vi "INIT_Q.vi"() -> (4 "MainQ Out":refnum<queue>, 6 "ACKQ Out":refnum<queue>, 8 "TempQ Out":refnum<queue>, 10 "MagQ Out":refnum<queue>, 15 "ScanQ Out":refnum<queue>)   [LabVIEW 2025]
uses:
  CTLs/Producer Cluster.ctl
  CTLs/ACK Cluster.ctl
  CTLs/TEMP CLUSTER.ctl
  CTLs/MAG CLUSTER.ctl
  CTLs/Scan Cluster.ctl
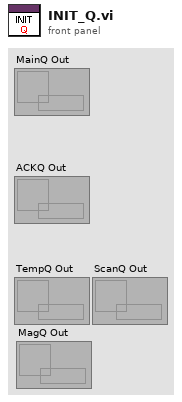
[diagram p1: front panel]
types:
  T1 = typedef "Scan Cluster.ctl" = cluster{"Setpoint (I)":dbl[], "Bias (V)":dbl[], "Number of scans":u8, "Port number (3364)":u32, "Avoid zero threshold (V)":dbl, "Current State":enum16{"1. BIAS", "2. SCAN", "3. SCAN_IDLE", "4. DRIFT CORRECT (SF)", "5. DRFT CORRECT (BS)", "6. STOP"}}
  T2 = typedef "MAG CLUSTER.ctl" = cluster{"Ramp Target":enum16{"ZERO", "MID", "MAX"}, "Pause":bool, "Switch Heater":bool, "Persistent Field":dbl, "Persistent Current":dbl, "Tesla":bool, "Output (T)":dbl, "Output (A)":dbl, "X Trip":enum16{"DISABLED", "ENABLED", "ACTIVE"}, "Ramp Rate (A/s)":dbl, "V Limit (V)":dbl, "Heater Voltage":dbl, "MAX Setpoint (A)":dbl, "MAX Setpoint (T)":dbl, "MID Setpoint (A)":dbl, "MID Setpoint (T)":dbl, "Lock":bool, "Field Constant":dbl, "Remote":bool, "Direction":enum16{"POSITIVE", "NEGATIVE", "OPEN", "UNIPOLAR"}, "Helium Level":u16, "Quench !":bool, "Voltage":dbl, "V Limit !":bool, "Ramping":bool, "At Target":bool, "Trip Field":dbl, "Trip Current":dbl, "Current State":enum16{"1. INIT MAG", "2. PREP FIELD", "3. APPLY FIELD", "4. MAG STAB", "5. MAG IDLE", "6. MAG OFF"}, "MAG Reference":refnum<visa-resource-name>}
  T3 = typedef "TEMP CLUSTER.ctl" = cluster{"Range (0:Off)":u16, "Manual Output (0.00 %)":dbl, "Rate (D) (0.0 %)":dbl, "Reset (I) (20.0)":dbl, "Gain (P) (50.0)":dbl, "Power Up Enable (F: Disable)":bool, "Max User Current (2.000)":dbl, "Heater Resistance (1:25 Ohms)":u16, "Max Current (0:User Specified)":u16, "Heater Out Display (1:Current)":u16, "Mode (0:Off)":u16, "Input (0:None)":u16, "Target Temp (K)":dbl, "Serial Configuration":cluster{"Baud Rate":u32, "Parity":u16, "Data Bits":u16, "Stop Bits":u16, "Flow Control":u16}, "VISA resource name":refnum<visa-resource-name>, "Configure Control Parameters (0: Configure)":u16, "Enable Setpoint (F:Disable)":bool, "Input (0:A)":u16, "Data Source (0:Kelvin)":u16, "Output's Control Loop (1:1)":u16, "STND DEV Threshold ":dbl, "Mean Tolerance ":dbl, "Current State":enum16{"1. INIT_TEMP", "2. SET_TEMP", "3. WAIT_STABLE", "4. TEMP_IDLE", "5. TC OFF (Reset)"}}
  T4 = typedef "ACK Cluster.ctl" = cluster{"ACK States":enum16{"1. TEMP STABLE", "2. FIELD STABLE", "3. SCAN DONE", "4. BIAS DONE", "5. DRIFT CORRECTED (SF)", "6. DRIFT CORRECTED (BS)"}, "Drift Correction Values":dbl[][]}
  T5 = typedef "Producer Cluster.ctl" = cluster{"Producer State":enum16{"1. INIT", "2. SET TEMP", "3. WAIT FOR STABILITY (T)", "4. SET FIELD ", "5. WAIT FOR STABILITY (B)", "6. RUN SCAN", "7. RUN BIAS", "8. DRIFT CORRECT (SF)", "9. DRIFT CORRECT (BS)", "10. ADVANCE", "11. SHUTDOWN"}, "Experiment Mode":enum16{"1. SWEEP FIELD", "2. SWEEP TEMP", "3. SWEEP FIELD AND TEMP"}, "Target Temp (K)":dbl[], "Target Field (T)":dbl[], "Temp Index":i32, "Field Index":i32, "Current Temp":dbl, "Current Field":dbl}
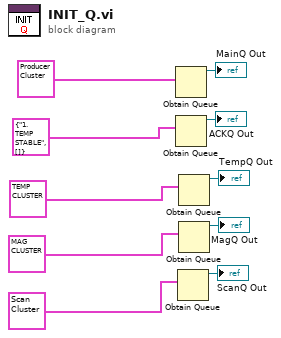
[diagram p0: block diagram]
diagram:
  n1 = Obtain Queue(element data type=T5 {"Producer State"=enum."1. INIT", "Experiment Mode"=enum."1. SWEEP FIELD", "Target Temp (K)"=[], "Target Field (T)"=[], "Temp Index"=0, "Field Index"=0, "Current Temp"=0.0, "Current Field"=0.0} ("Producer Cluster")) -> (queue out=→"MainQ Out":refnum<queue>)  [unwired: 4 in, 2 out]
  n2 = Obtain Queue(element data type=T4 {"ACK States"=enum."1. TEMP STABLE", "Drift Correction Values"=[]} ("ACK Cluster")) -> (queue out=→"ACKQ Out":refnum<queue>)  [unwired: 4 in, 2 out]
  n3 = Obtain Queue(element data type=T1 {"Setpoint (I)"=[], "Bias (V)"=[], "Number of scans"=1, "Port number (3364)"=3364, "Avoid zero threshold (V)"=0.004999999888241291, "Current State"=enum."1. BIAS"} ("Scan Parameters")) -> (queue out=→"ScanQ Out":refnum<queue>)  [unwired: 4 in, 2 out]
  n4 = Obtain Queue(element data type=T3 {"Range (0:Off)"=0, "Manual Output (0.00 %)"=0.0, "Rate (D) (0.0 %)"=0.0, "Reset (I) (20.0)"=20.0, "Gain (P) (50.0)"=50.0, "Power Up Enable (F: Disable)"=FALSE, "Max User Current (2.000)"=2.0, "Heater Resistance (1:25 Ohms)"=1, "Max Current (0:User Specified)"=0, "Heater Out Display (1:Current)"=1, "Mode (0:Off)"=1, "Input (0:None)"=4, "Target Temp (K)"=5.0, "Serial Configuration"={"Baud Rate"=57600, "Parity"=1, "Data Bits"=7, "Stop Bits"=10, "Flow Control"=0}, "VISA resource name"="", "Configure Control Parameters (0: Configure)"=0, "Enable Setpoint (F:Disable)"=FALSE, "Input (0:A)"=3, "Data Source (0:Kelvin)"=0, "Output's Control Loop (1:1)"=2, "STND DEV Threshold "=0.1, "Mean Tolerance "=0.01, "Current State"=enum."1. INIT_TEMP"} ("Temp Controller")) -> (queue out=→"TempQ Out":refnum<queue>)  [unwired: 4 in, 2 out]
  n5 = Obtain Queue(element data type=T2 {"Ramp Target"=enum."ZERO", "Pause"=FALSE, "Switch Heater"=FALSE, "Persistent Field"=0.0, "Persistent Current"=0.0, "Tesla"=FALSE, "Output (T)"=0.0, "Output (A)"=0.0, "X Trip"=enum."DISABLED", "Ramp Rate (A/s)"=0.0, "V Limit (V)"=0.0, "Heater Voltage"=0.0, "MAX Setpoint (A)"=0.0, "MAX Setpoint (T)"=0.0, "MID Setpoint (A)"=0.0, "MID Setpoint (T)"=0.0, "Lock"=FALSE, "Field Constant"=0.0, "Remote"=FALSE, "Direction"=enum."POSITIVE", "Helium Level"=0, "Quench !"=FALSE, "Voltage"=0.0, "V Limit !"=FALSE, "Ramping"=FALSE, "At Target"=FALSE, "Trip Field"=0.0, "Trip Current"=0.0, "Current State"=enum."1. INIT MAG", "MAG Reference"="COM4"} ("PSU Status In")) -> (queue out=→"MagQ Out":refnum<queue>)  [unwired: 4 in, 2 out]
